vi "Get.vi"(8 "error in (no error)":errorcluster, 11 "Variant DVR in":refnum<data-value>) -> (0 "error out":errorcluster, 2 "Variant":variant, 3 "Variant DVR out":refnum<data-value>)   [LabVIEW 2019, in "Variant Attributes.lvlib"]
uses:
  Variant Attributes.lvlib
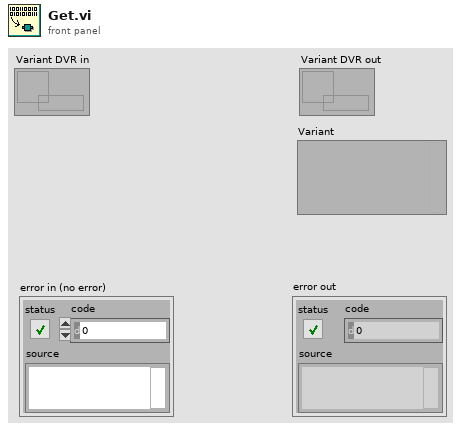
[diagram p1: front panel]
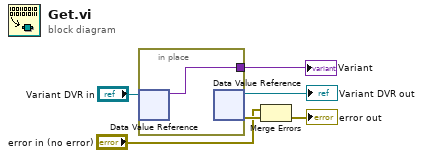
[diagram p0: block diagram]
diagram:
  n1 = in-place {
    in-place-border: [w7] -> w1
    n2 = in-place-dvr #1("Variant DVR in") -> (w7:variant)  [unwired: 1 out]
    n3 = in-place-dvr #1() -> (→"Variant DVR out":refnum<data-value>, w4:errorcluster)  [unwired: 1 in]
  }
  "Variant" <- w1
  n4 = Merge Errors("error in (no error)", w4) -> (→"error out":errorcluster)
